vi "LabView_main.vi"() -> ()   [LabVIEW 2019]
panel:
  out "return value 2":dbl[](array[numeric])
  out "return value":dbl
  in  "In1 3":dbl
  in  "In1 2":dbl
  in  "In1":dbl
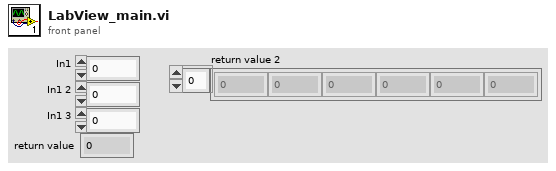
[diagram p1: front panel]
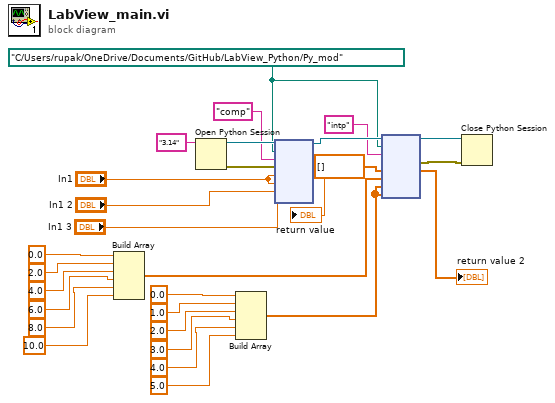
[diagram p0: block diagram]
diagram:
  w20 = path "C:/Users/rupak/OneDrive/Documents/GitHub/LabView_Python/Py_mod" ("module path")
  n1 = Build Array(0.0 ("element"), 2.0 ("element"), 4.0 ("element"), 6.0 ("element"), 8.0 ("element"), 10.0 ("element")) -> (w14:dbl[])
  n2 = Open Python Session(python version="3.14" ("Python version")) -> (session out=w28:refnum<k35>, error out=w27:errorcluster)  [unwired: 2 in]
  n3 = Build Array(0.0 ("element"), 1.0 ("element"), 2.0 ("element"), 3.0 ("element"), 4.0 ("element"), 5.0 ("element")) -> (w1:dbl[])
  n4 = node(w28, w20, "comp" ("function name"), w27, "In1", "In1", "In1 2", "In1 3") -> (w21:refnum<k35>, →"return value":dbl)  [unwired: 3 in, 3 out]
  n5 = node(w21, w20, "intp" ("function name"), dbl[] [] ("appended array"), w14, w1, w1) -> (w16:refnum<k35>, w15:errorcluster, →"return value 2":dbl[])  [unwired: 4 in, 2 out]
  n6 = Close Python Session(session in=w16, error in=w15) -> ()  [unwired: 1 out]
